vi "Reset.vi"(8 "error in (no error)":errorcluster, 11 "VISA resource name":refnum<visa-resource-name>) -> (0 "error out":errorcluster, 3 "VISA resource name out":refnum<visa-resource-name>)   [LabVIEW 2020, in "IT6500.lvlib"]
doc: "Resets the instrument and then sends a set of default setup commands to the instrument."
uses:
  IT6500.lvlib
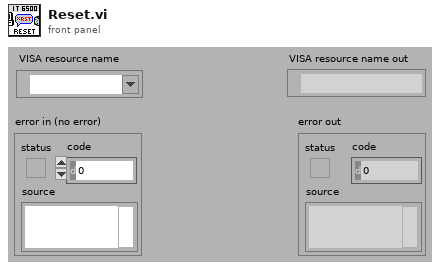
[diagram p1: front panel]
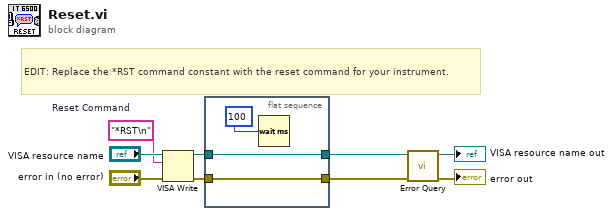
[diagram p0: block diagram]
diagram:
  w7 = "*RST\n"  # Reset Command
  # "EDIT: Replace the *RST command constant with the reset command for your instrument."
  n1 = VISA Write(VISA resource name="VISA resource name", write buffer=w7, error in (no error)="error in (no error)") -> (VISA resource name out=w4:refnum<visa-resource-name>, error out=w3:errorcluster)  [unwired: 1 out]
  n2 = flat-sequence {
    tunnel: w4 -> [w11]
    tunnel: w3 -> [w10]
    tunnel: [w11] -> w2
    tunnel: [w10] -> w1
    frame #0 {
      n3 = Wait (ms)(milliseconds to wait=100) -> ()  [unwired: 1 out]
    }
  }
  n4 = call "Error Query.vi"("error in (no error)"=w1, "VISA resource name"=w2) -> ("error out"=→"error out":errorcluster, "VISA resource name out"=→"VISA resource name out":refnum<visa-resource-name>)  [unwired: 6 in, 2 out]
